vi "Variant to Datatype.vi"(10 "error in":errorcluster, 11 "Variant":variant) -> (2 "error out":errorcluster, 3 "DataType":refnum<class "GDSII.DataType.lvclass">)   [LabVIEW 2019, in "GDSII.DataType.lvclass"]
uses:
  GDSII.DataType.lvclass
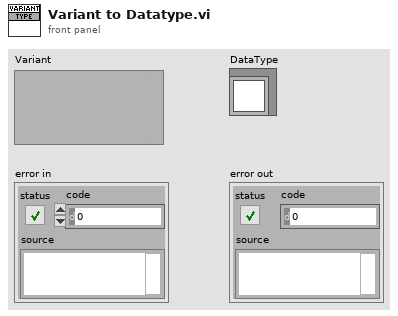
[diagram p1: front panel]
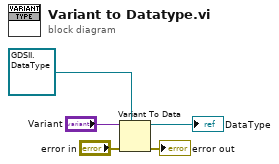
[diagram p0: block diagram]
diagram:
  n1 = Variant To Data(error in="error in", type=refnum<class "GDSII.DataType.lvclass"> refnum ("GDSII.DataType.lvclass"), Variant="Variant") -> (data=→"DataType":refnum<class "GDSII.DataType.lvclass">, error out=→"error out":errorcluster)
